vi "Populate Result.vi"(8 "error in (no error)":errorcluster, 11 "Step in":refnum<class "Step.lvclass">) -> (0 "error out":errorcluster, 3 "Step out":refnum<class "Step.lvclass">)   [LabVIEW 2015, in "Step.lvclass"]
doc: "This VI Gathers the information from the step and builds a result with it."
uses:
  Step.lvclass
  Step.lvclass/Step.ctl
  Result/Result.lvclass
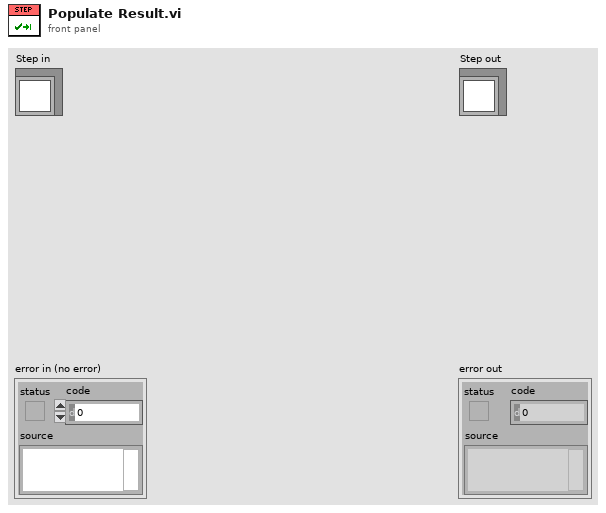
[diagram p1: front panel]
types:
  T1 = typedef "Step.lvclass/Step Status.ctl" = enum16{"Start", "Passed", "Failed", "Error", "Done", "Terminated", "Skipped", "Running"}
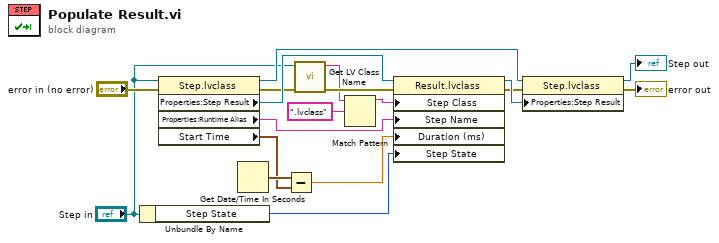
[diagram p0: block diagram]
diagram:
  n1 = Unbundle By Name("Step in") -> ("Step State"=w1:T1)
  n2 = property class="Step.lvclass"(reference="Step in", error in="error in (no error)") -> (reference out=w16:refnum<class "Step.lvclass">, error out=w11:errorcluster, "Properties:Step Result"=w15:refnum<class "Result.lvclass">, "Properties:Runtime Alias"=w9:string, "Start Time"=w7:timestamp)
  n3 = Get Date/Time In Seconds() -> (seconds since 1Jan1904=w8:timestamp)
  n4 = Subtract(x=w8, y=w7) -> (x-y=w6:dbl)
  n5 = call <vilib>:"Get LV Class Name.vi"("error in (no error)"=w11, "object"="Step in") -> ("error out"=w10:errorcluster, "class name"=w5:string)  [unwired: 8 in]
  n6 = Match Pattern(string=w5, regular expression=".lvclass") -> (before substring=w3:string)  [unwired: 1 in, 3 out]
  n7 = property class="Result.lvclass"(reference=w15, error in=w10, "Step Class"=w3, "Step Name"=w9, "Duration (ms)"=w6, "Step State"=w1) -> (reference out=w14:refnum<class "Result.lvclass">, error out=w13:errorcluster)
  n8 = property class="Step.lvclass"(reference=w16, error in=w13, "Properties:Step Result"=w14) -> (reference out=→"Step out":refnum<class "Step.lvclass">, error out=→"error out":errorcluster)
